vi "Read Results.vi"(8 "error in (no error)":errorcluster, 11 "Combined Result in":refnum<class "Combined Result.lvclass">) -> (0 "error out":errorcluster, 2 "Results":refnum<class "Acquired Result.lvclass">[](array[class]), 3 "Combined Result out":refnum<class "Combined Result.lvclass">)   [LabVIEW 2021, in "Combined Result.lvclass"]
uses:
  Combined Result.lvclass
  Acquired Result/Acquired Result.lvclass
  Combined Result.lvclass/Combined Result.ctl
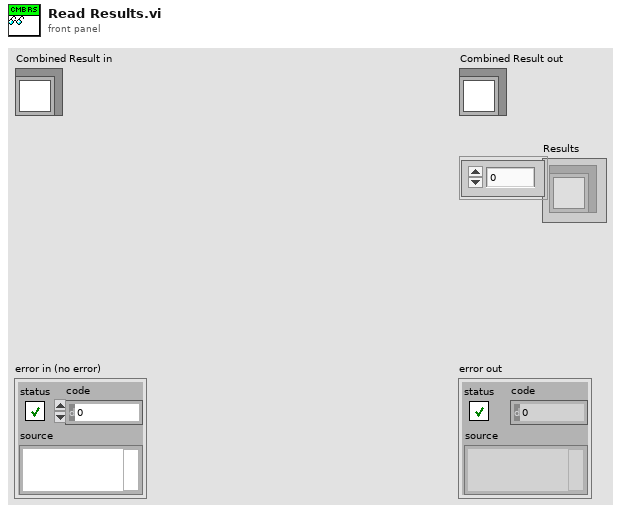
[diagram p1: front panel]
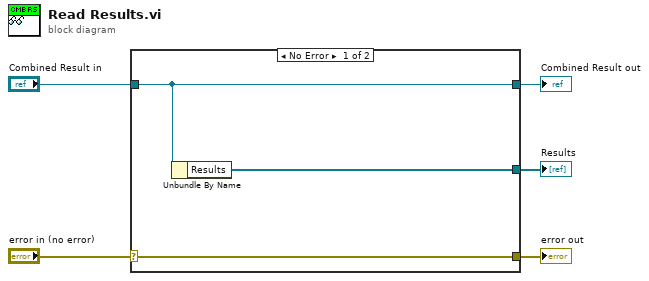
[diagram p0: block diagram]
diagram:
  n1 = case shown="No Error" "error in (no error)" {
    selector: "error in (no error)" -> [w8 w9]
    tunnel: [w8 w9] -> w4
    tunnel: [w7 w10] -> w2
    tunnel: "Combined Result in" -> [w7 w10]
    tunnel: [w6 _] -> w1
    frame No Error {
      n2 = Unbundle By Name(w7) -> ("Results"=w6:refnum<class "Acquired Result.lvclass">[])
    }
    frame Error {
    }
  }
  "error out" <- w4
  "Combined Result out" <- w2
  "Results" <- w1
